vi "Teleop.vi"(10 "Match Info":T1={"Autonomous Elapsed Seconds"=0.0, "TeleOp Elapsed Seconds"=0.0, "Disabled Elapsed Seconds"=0.0, "Visited Autonomous"=FALSE, "Visited TeleOp"=FALSE, "Visited Disabled"=FALSE, "Autonomous Settings"={"Autonomous Style"=enum."Independent", "VI Refnum"=refnum}}, 11 "Call Context":T2) -> ()   [LabVIEW 2019]
doc: "This VI is called for each TeleOp packet received from the DS where the robot is not disabled. It is often used to read from the joysticks and update I/O or to update setpoints for timed control loops. It should complete and return within 20 milliseconds or it may miss DS packets."
uses:
  <vilib>/Rock Robotics/WPI/DriverStation/WPI_DriverStationDerivedRobotMode.ctl
  <vilib>/Rock Robotics/WPI/DriverStation/WPI_DriverStationMatch Info.ctl
  <vilib>/Rock Robotics/WPI/Utilities/WPI_GetSetVariantRefNum.vi
  Robot Global Data.vi
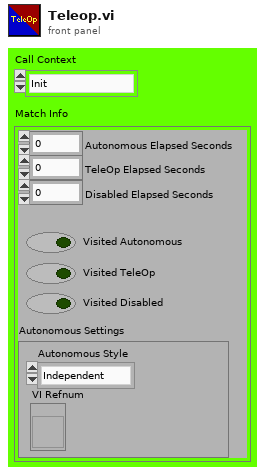
[diagram p1: front panel]
types:
  T1 = typedef "WPI_DriverStationMatch Info.ctl" = cluster{"Autonomous Elapsed Seconds":dbl, "TeleOp Elapsed Seconds":dbl, "Disabled Elapsed Seconds":dbl, "Visited Autonomous":bool, "Visited TeleOp":bool, "Visited Disabled":bool, "Autonomous Settings":cluster{"Autonomous Style":enum16{"Iterative", "Independent"}, "VI Refnum":refnum<vi>}}
  T2 = typedef "WPI_DriverStationDerivedRobotMode.ctl" = enum16{"Init", "Execute", "Stop"}
  T3 = typedef "WPI_JoystickDevRef.ctl" = cluster{"Device":T4}
  T4 = typedef "WPI_JoystickDeviceEnum.ctl" = enum16{"USB 0", "USB 1", "USB 2", "USB 3", "USB 4", "USB 5"}
  T5 = cluster{"Axes[0]":dbl, "Axes[1]":dbl, "Axes[2]":dbl, "Axes[3]":dbl, "Axes[4]":dbl, "Axes[5]":dbl, "Axes[6]":dbl, "Axes[7]":dbl}
  T6 = cluster{"Buttons[0]":bool, "Buttons[1]":bool, "Buttons[2]":bool, "Buttons[3]":bool, "Buttons[4]":bool, "Buttons[5]":bool, "Buttons[6]":bool, "Buttons[7]":bool, "Buttons[8]":bool, "Buttons[9]":bool, "Buttons[10]":bool, "Buttons[11]":bool, "Buttons[12]":bool, "Buttons[13]":bool, "Buttons[14]":bool, "Buttons[15]":bool, "Buttons[16]":bool, "Buttons[17]":bool, "Buttons[18]":bool, "Buttons[19]":bool, "Buttons[20]":bool, "Buttons[21]":bool, "Buttons[22]":bool, "Buttons[23]":bool, "Buttons[24]":bool, "Buttons[25]":bool, "Buttons[26]":bool, "Buttons[27]":bool, "Buttons[28]":bool, "Buttons[29]":bool, "Buttons[30]":bool, "Buttons[31]":bool, "Buttons[32]":bool, "Buttons[33]":bool, "Buttons[34]":bool, "Buttons[35]":bool, "Buttons[36]":bool, "Buttons[37]":bool, "Buttons[38]":bool, "Buttons[39]":bool, "Buttons[40]":bool, "Buttons[41]":bool, "Buttons[42]":bool, "Buttons[43]":bool, "Buttons[44]":bool, "Buttons[45]":bool, "Buttons[46]":bool, "Buttons[47]":bool, "Buttons[48]":bool, "Buttons[49]":bool}
  T7 = cluster{"POVs[0]":i16, "POVs[1]":i16, "POVs[2]":i16, "POVs[3]":i16, "POVs[4]":i16, "POVs[5]":i16, "POVs[6]":i16, "POVs[7]":i16, "POVs[8]":i16}
  T8 = cluster{"A1":dbl, "A2":dbl, "A3":dbl, "A4":dbl, "A5":dbl, "A6":dbl, "A7":dbl, "A8":dbl}
  T9 = cluster{"1":bool, "2":bool, "3":bool, "4":bool, "5":bool, "6":bool, "7":bool, "8":bool, "9":bool, "10":bool, "11":bool, "12":bool, "13":bool, "14":bool, "15":bool, "16":bool, "17":bool, "18":bool, "19":bool, "20":bool, "21":bool, "22":bool, "23":bool, "24":bool, "25":bool, "26":bool, "27":bool, "28":bool, "29":bool, "30":bool, "31":bool, "32":bool, "33":bool, "34":bool, "35":bool, "36":bool, "37":bool, "38":bool, "39":bool, "40":bool, "41":bool, "42":bool, "43":bool, "44":bool, "45":bool, "46":bool, "47":bool, "48":bool, "49":bool, "50":bool}
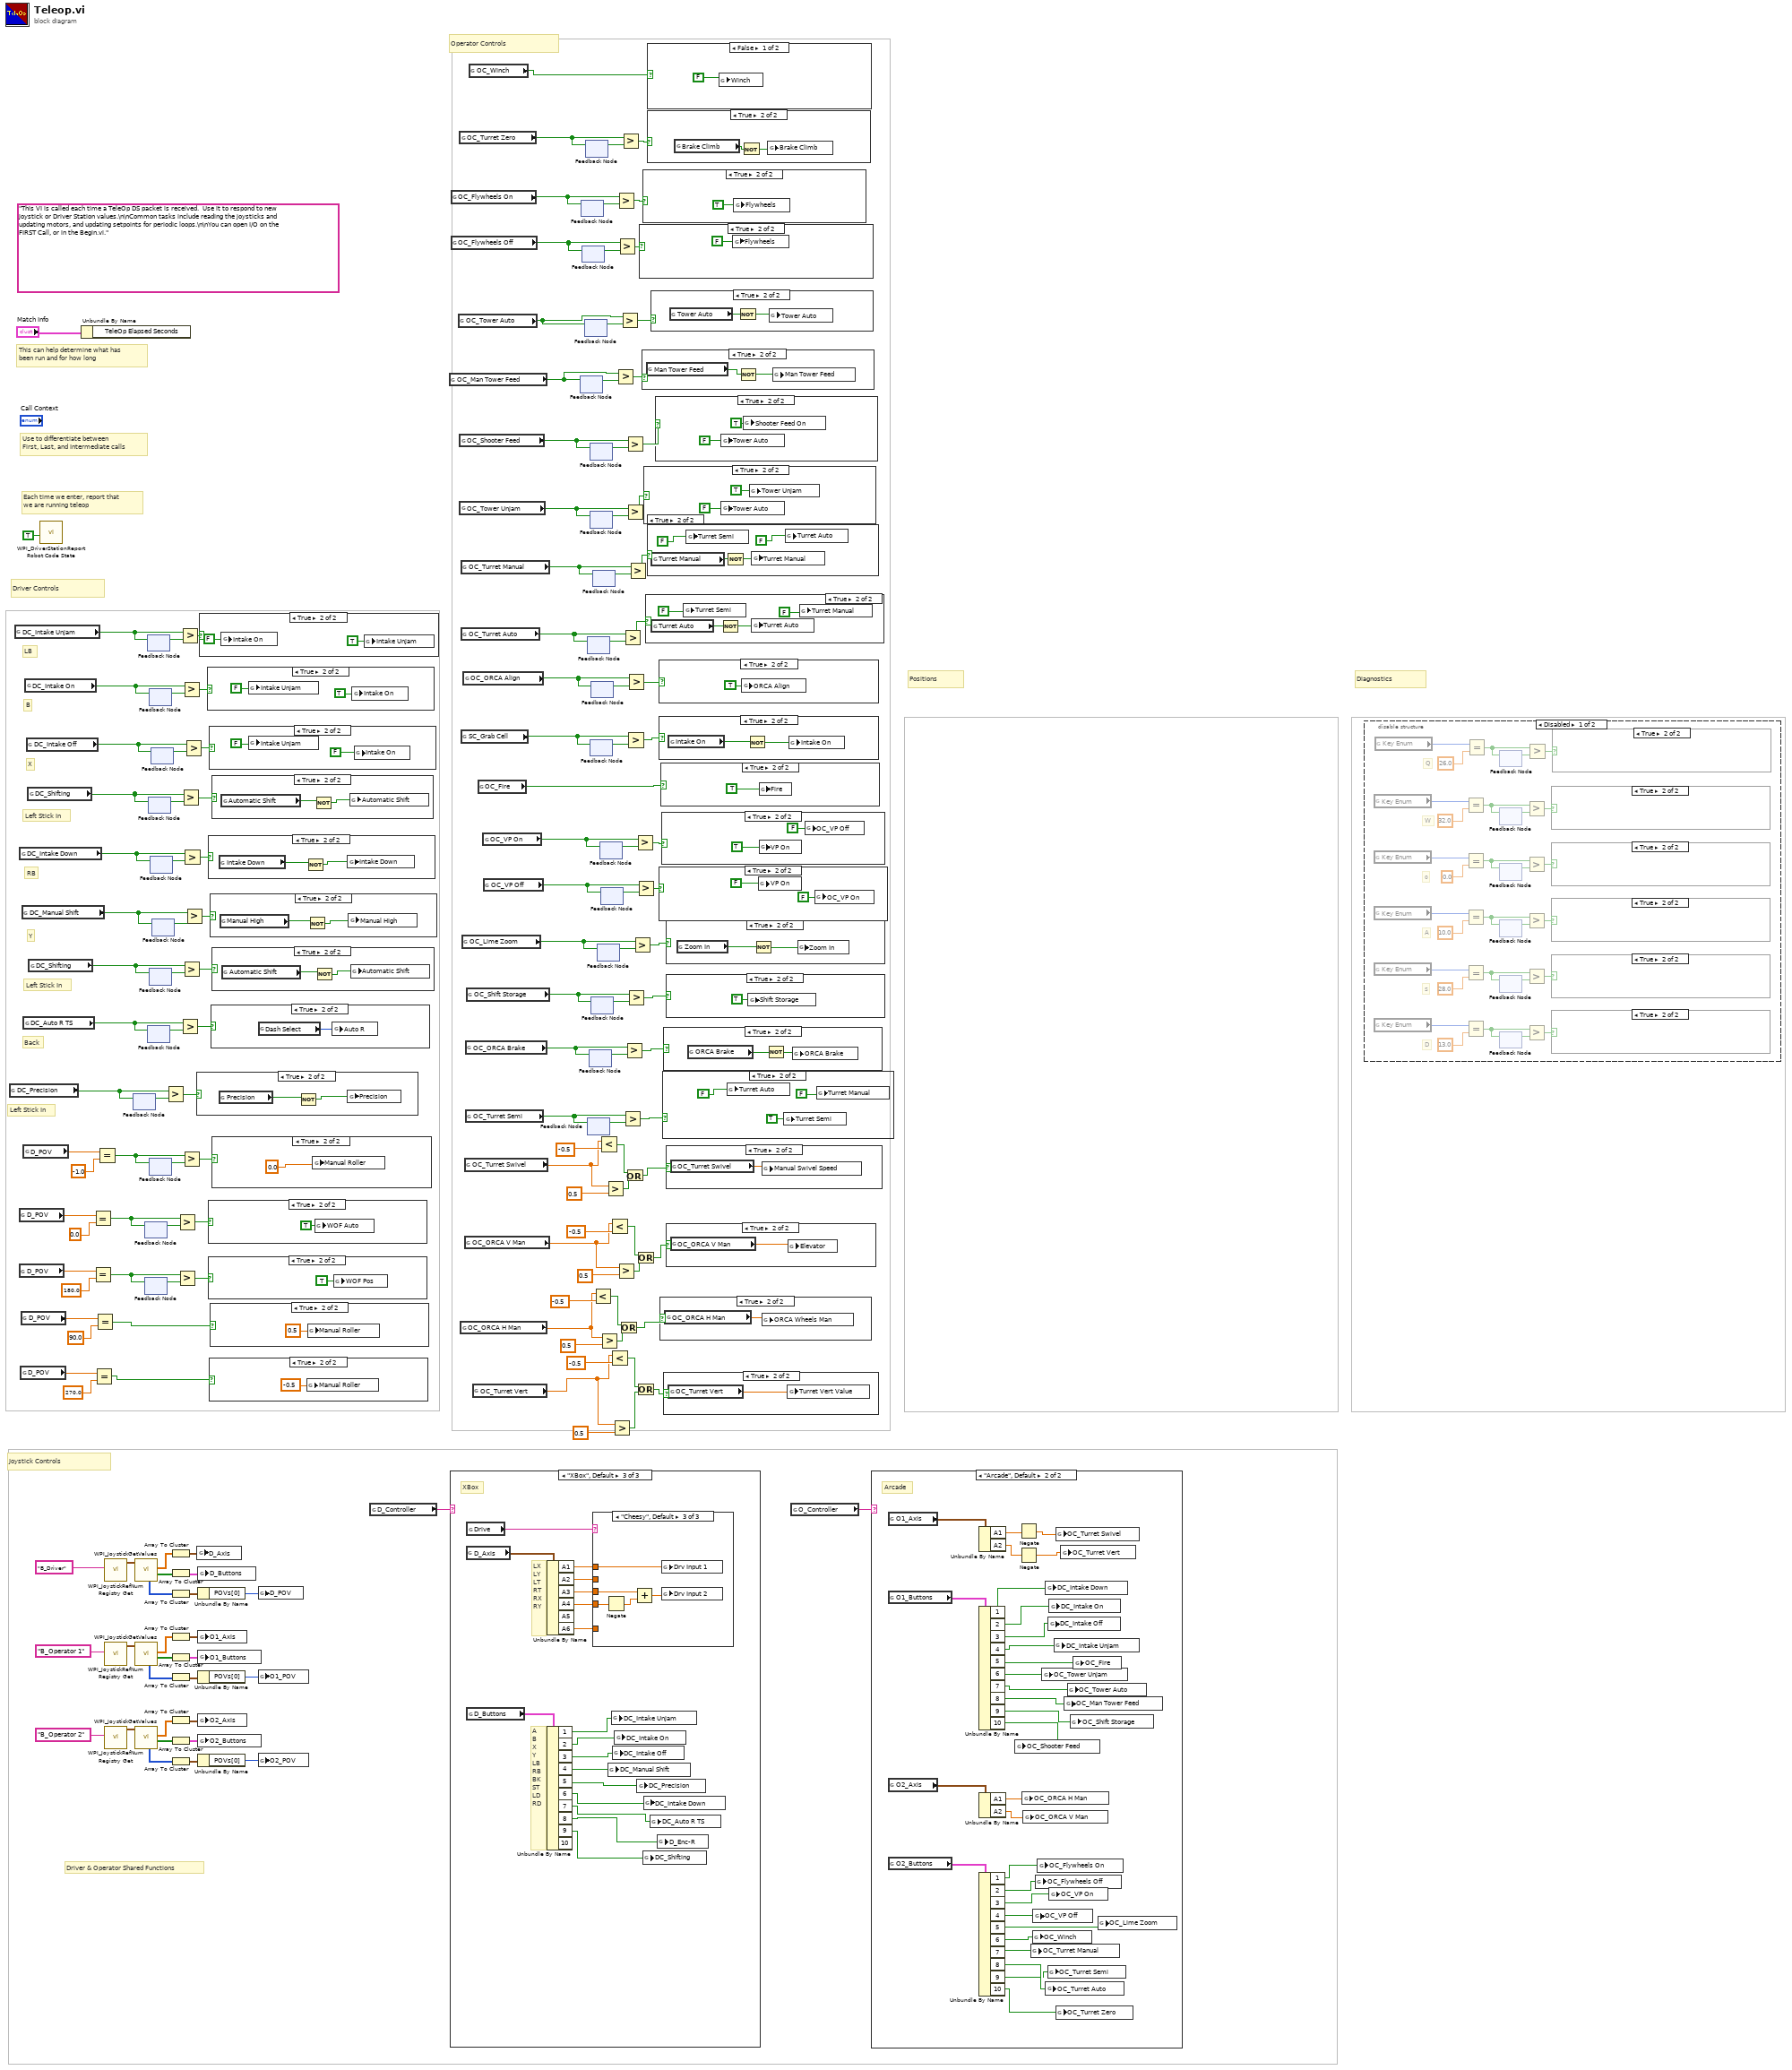
[diagram p0: block diagram]
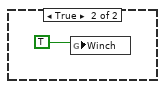
[diagram p2: hidden frame]
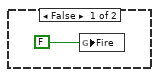
[diagram p7: hidden frame]
diagram:
  (unwired) "This VI is called each time a TeleOp DS packet is received.  Use it to respond to new joystick or Driver Station values.\n\nCommon tasks include reading the joysticks and updating motors, and updating setpoints for periodic loops.\n\nYou can open I/O on the FIRST Call, or in the Begin.vi."
  # "Left Stick In"
  # "B"
  # "X"
  # "Left Stick In"
  # "RB"
  # "Y"
  # "Left Stick In"
  # "Driver & Operator Shared Functions"
  # "Joystick Controls"
  # "Positions"
  # "Diagnostics"
  # "Operator Controls"
  # "Back"
  # "LB"
  # "Driver Controls"
  # "Each time we enter, report that\nwe are running teleop"
  # "Use to differentiate between\nFirst, Last, and Intermediate calls"
  # "This can help determine what has\nbeen run and for how long"
  n1 = global read "Robot Global Data.vi" "DC_Precision"() -> (w7:bool)
  n2 = global read "Robot Global Data.vi" "DC_Intake Unjam"() -> (w143:bool)
  n3 = global read "Robot Global Data.vi" "D_POV"() -> (w138:dbl)
  n4 = global read "Robot Global Data.vi" "D_POV"() -> (w148:dbl)
  n5 = global read "Robot Global Data.vi" "DC_Intake Down"() -> (w71:bool)
  n6 = global read "Robot Global Data.vi" "D_POV"() -> (w154:dbl)
  n7 = global read "Robot Global Data.vi" "D_POV"() -> (w84:dbl)
  n8 = global read "Robot Global Data.vi" "DC_Manual Shift"() -> (w76:bool)
  n9 = global read "Robot Global Data.vi" "DC_Auto R TS"() -> (w152:bool)
  n10 = global read "Robot Global Data.vi" "D_POV"() -> (w80:dbl)
  n11 = global read "Robot Global Data.vi" "DC_Intake On"() -> (w70:bool)
  n12 = global read "Robot Global Data.vi" "DC_Intake Off"() -> (w65:bool)
  n13 = global read "Robot Global Data.vi" "DC_Shifting"() -> (w64:bool)
  n14 = global read "Robot Global Data.vi" "DC_Shifting"() -> (w86:bool)
  n15 = call <vilib>:"WPI_DriverStationReport Robot Code State.vi"("TeleOp"=TRUE ("Autonomous")) -> ()  [unwired: 10 in, 1 out]
  n16 = Unbundle By Name("Match Info") -> ()  [unwired: 1 out]
  n17 = Equal?(x=w138, y=0.0) -> (x = y?=w144:bool)
  n18 = Equal?(x=w148, y=180.0) -> (x = y?=w145:bool)
  n19 = Equal?(x=w154, y=270.0) -> (x = y?=w83:bool)
  n20 = Equal?(x=w84, y=90.0) -> (x = y?=w82:bool)
  n21 = Equal?(x=w80, y=-1.0) -> (x = y?=w77:bool)
  n22 = call <vilib>:"WPI_JoystickRefNum Registry Get.vi"("refnum name"="B_Driver") -> ("JoystickDevRef"=w136:T3)  [unwired: 9 in, 1 out]
  n23 = call <vilib>:"WPI_JoystickRefNum Registry Get.vi"("refnum name"="B_Operator 1") -> ("JoystickDevRef"=w122:T3)  [unwired: 9 in, 1 out]
  n24 = call <vilib>:"WPI_JoystickRefNum Registry Get.vi"("refnum name"="B_Operator 2") -> ("JoystickDevRef"=w119:T3)  [unwired: 9 in, 1 out]
  n25 = feedback #1() -> (w5:bool)  [unwired: 1 in]
  n26 = feedback-in #1(w7) -> ()
  n27 = call <vilib>:"WPI_JoystickGetValues.vi"("JoystickDevRef"=w136) -> ("Buttons"=w134:bool[], "Axes"=w133:dbl[], "POVs"=w132:i16[])  [unwired: 6 in, 2 out]
  n28 = call <vilib>:"WPI_JoystickGetValues.vi"("JoystickDevRef"=w122) -> ("Buttons"=w124:bool[], "Axes"=w125:dbl[], "POVs"=w126:i16[])  [unwired: 6 in, 2 out]
  n29 = call <vilib>:"WPI_JoystickGetValues.vi"("JoystickDevRef"=w119) -> ("Buttons"=w117:bool[], "Axes"=w116:dbl[], "POVs"=w115:i16[])  [unwired: 6 in, 2 out]
  n30 = feedback #2() -> (w141:bool)  [unwired: 1 in]
  n31 = feedback-in #2(w144) -> ()
  n32 = feedback #3() -> (w147:bool)  [unwired: 1 in]
  n33 = feedback-in #3(w145) -> ()
  n34 = feedback #4() -> (w139:bool)  [unwired: 1 in]
  n35 = feedback-in #4(w143) -> ()
  n36 = feedback #5() -> (w150:bool)  [unwired: 1 in]
  n37 = feedback-in #5(w152) -> ()
  n38 = feedback #6() -> (w62:bool)  [unwired: 1 in]
  n39 = feedback-in #6(w64) -> ()
  n40 = feedback #7() -> (w68:bool)  [unwired: 1 in]
  n41 = feedback-in #7(w70) -> ()
  n42 = feedback #8() -> (w88:bool)  [unwired: 1 in]
  n43 = feedback-in #8(w86) -> ()
  n44 = feedback #9() -> (w79:bool)  [unwired: 1 in]
  n45 = feedback-in #9(w77) -> ()
  n46 = feedback #10() -> (w73:bool)  [unwired: 1 in]
  n47 = feedback-in #10(w71) -> ()
  n48 = feedback #11() -> (w67:bool)  [unwired: 1 in]
  n49 = feedback-in #11(w65) -> ()
  n50 = feedback #12() -> (w74:bool)  [unwired: 1 in]
  n51 = feedback-in #12(w76) -> ()
  n52 = Greater?(x=w7, y=w5) -> (0:w6:bool)
  n53 = Array To Cluster(array=w133) -> (cluster=w130:T5)
  n54 = Array To Cluster(array=w134) -> (cluster=w129:T6)
  n55 = Array To Cluster(array=w132) -> (cluster=w131:T7)
  n56 = Array To Cluster(array=w125) -> (cluster=w121:T5)
  n57 = Array To Cluster(array=w124) -> (cluster=w128:T6)
  n58 = Array To Cluster(array=w126) -> (cluster=w127:T7)
  n59 = Array To Cluster(array=w116) -> (cluster=w120:T5)
  n60 = Array To Cluster(array=w117) -> (cluster=w113:T6)
  n61 = Array To Cluster(array=w115) -> (cluster=w114:T7)
  n62 = Greater?(x=w144, y=w141) -> (0:w142:bool)
  n63 = Greater?(x=w145, y=w147) -> (0:w146:bool)
  n64 = Greater?(x=w143, y=w139) -> (0:w140:bool)
  n65 = Greater?(x=w152, y=w150) -> (0:w151:bool)
  n66 = Greater?(x=w64, y=w62) -> (0:w63:bool)
  n67 = Greater?(x=w70, y=w68) -> (0:w69:bool)
  n68 = Greater?(x=w86, y=w88) -> (0:w87:bool)
  n69 = Greater?(x=w77, y=w79) -> (0:w78:bool)
  n70 = Greater?(x=w71, y=w73) -> (0:w72:bool)
  n71 = Greater?(x=w65, y=w67) -> (0:w66:bool)
  n72 = Greater?(x=w76, y=w74) -> (0:w75:bool)
  n73 = case shown="True" w6 {
    frame False {
    }
    frame True {
      n74 = global read "Robot Global Data.vi" "Precision"() -> (w158:bool)
      n75 = Not(x=w158) -> (.not. x?=w157:bool)
      n76 = global write "Robot Global Data.vi" "Precision"(w157) -> ()
    }
  }
  n77 = global write "Robot Global Data.vi" "D_Axis"(w130) -> ()
  n78 = global write "Robot Global Data.vi" "D_Buttons"(w129) -> ()
  n79 = Unbundle By Name(w131) -> ("POVs[0]"=w112:i16)
  n80 = global write "Robot Global Data.vi" "O1_Axis"(w121) -> ()
  n81 = global write "Robot Global Data.vi" "O1_Buttons"(w128) -> ()
  n82 = Unbundle By Name(w127) -> ("POVs[0]"=w111:i16)
  n83 = global write "Robot Global Data.vi" "O2_Axis"(w120) -> ()
  n84 = global write "Robot Global Data.vi" "O2_Buttons"(w113) -> ()
  n85 = Unbundle By Name(w114) -> ("POVs[0]"=w110:i16)
  n86 = case shown="True" w140 {
    frame False {
    }
    frame True {
      n87 = global write "Robot Global Data.vi" "Intake On"(FALSE ("Intake On")) -> ()
      n88 = global write "Robot Global Data.vi" "Intake Unjam"(TRUE ("Intake Unjam")) -> ()
    }
  }
  n89 = case shown="True" w69 {
    frame False {
    }
    frame True {
      n90 = global write "Robot Global Data.vi" "Intake Unjam"(FALSE ("Intake On")) -> ()
      n91 = global write "Robot Global Data.vi" "Intake On"(TRUE ("Intake On")) -> ()
    }
  }
  n92 = case shown="True" w72 {
    frame False {
    }
    frame True {
      n93 = global read "Robot Global Data.vi" "Intake Down"() -> (w164:bool)
      n94 = Not(x=w164) -> (.not. x?=w163:bool)
      n95 = global write "Robot Global Data.vi" "Intake Down"(w163) -> ()
    }
  }
  n96 = case shown="True" w142 {
    frame False {
    }
    frame True {
      n97 = global write "Robot Global Data.vi" "WOF Auto"(TRUE ("DC_WOF")) -> ()
    }
  }
  n98 = case shown="True" w146 {
    frame False {
    }
    frame True {
      n99 = global write "Robot Global Data.vi" "WOF Pos"(TRUE ("WOF Pos")) -> ()
    }
  }
  n100 = case shown="True" w66 {
    frame False {
    }
    frame True {
      n101 = global write "Robot Global Data.vi" "Intake Unjam"(FALSE ("Intake On")) -> ()
      n102 = global write "Robot Global Data.vi" "Intake On"(FALSE ("Manual High")) -> ()
    }
  }
  n103 = case shown="True" w83 {
    frame False {
    }
    frame True {
      n104 = global write "Robot Global Data.vi" "Manual Roller"(-0.5 ("Manual Roller")) -> ()
    }
  }
  n105 = case shown="True" w75 {
    frame False {
    }
    frame True {
      n106 = global read "Robot Global Data.vi" "Manual High"() -> (w171:bool)
      n107 = Not(x=w171) -> (.not. x?=w170:bool)
      n108 = global write "Robot Global Data.vi" "Manual High"(w170) -> ()
    }
  }
  n109 = case shown="True" w82 {
    frame False {
    }
    frame True {
      n110 = global write "Robot Global Data.vi" "Manual Roller"(0.5 ("Manual Roller")) -> ()
    }
  }
  n111 = case shown="True" w151 {
    frame False {
    }
    frame True {
      n112 = global read "Robot Global Data.vi" "Dash Select"() -> (w173:i8)
      n113 = global write "Robot Global Data.vi" "Auto R"(w173) -> ()
    }
  }
  n114 = case shown="True" w63 {
    frame False {
    }
    frame True {
      n115 = global read "Robot Global Data.vi" "Automatic Shift"() -> (w175:bool)
      n116 = Not(x=w175) -> (.not. x?=w174:bool)
      n117 = global write "Robot Global Data.vi" "Automatic Shift"(w174) -> ()
    }
  }
  n118 = case shown="True" w87 {
    frame False {
    }
    frame True {
      n119 = global read "Robot Global Data.vi" "Automatic Shift"() -> (w177:bool)
      n120 = Not(x=w177) -> (.not. x?=w176:bool)
      n121 = global write "Robot Global Data.vi" "Automatic Shift"(w176) -> ()
    }
  }
  n122 = case shown="True" w78 {
    frame False {
    }
    frame True {
      n123 = global write "Robot Global Data.vi" "Manual Roller"(0.0 ("Manual Roller")) -> ()
    }
  }
  n124 = global write "Robot Global Data.vi" "D_POV"(w112) -> ()
  n125 = global write "Robot Global Data.vi" "O1_POV"(w111) -> ()
  n126 = global write "Robot Global Data.vi" "O2_POV"(w110) -> ()
  n127 = global read "Robot Global Data.vi" "D_Controller"() -> (w109:string)
  n128 = global read "Robot Global Data.vi" "OC_Man Tower Feed"() -> (w3:bool)
  n129 = case shown="\"XBox\", Default" w109 {
    frame "Sticks" {
    }
    frame "Steering" {
    }
    frame "XBox", Default {
      # "LX\nLY\nLT\nRT\nRX\nRY"
      # "A\nB\nX\nY\nLB\nRB\nBK\nST\nLD\nRD"
      # "XBox"
      n130 = global read "Robot Global Data.vi" "D_Axis"() -> (w195:T8)
      n131 = global read "Robot Global Data.vi" "Drive"() -> (w194:string)
      n132 = global read "Robot Global Data.vi" "D_Buttons"() -> (w188:T9)
      n133 = Unbundle By Name(w195) -> ("A1"=w193:dbl, "A2"=w190:dbl, "A3"=w192:dbl, "A4"=w191:dbl, "A6"=w189:dbl)  [unwired: 1 out]
      n134 = Unbundle By Name(w188) -> ("1"=w181:bool, "2"=w182:bool, "3"=w183:bool, "4"=w185:bool, "5"=w187:bool, "6"=w184:bool, "7"=w179:bool, "8"=w180:bool, "9"=w186:bool)  [unwired: 1 out]
      n135 = case shown="\"Cheesy\", Default" w194 {
        tunnel: w193 -> [_ w199 w204]
        tunnel: w192 -> [_ _ w203]
        tunnel: w191 -> [_ _ w202]
        tunnel: w190 -> [w197 w198 _]
        tunnel: w189 -> [w196 _ _]
        frame "Tank" {
          n136 = global write "Robot Global Data.vi" "Drv Input 1"(w197) -> ()
          n137 = global write "Robot Global Data.vi" "Drv Input 2"(w196) -> ()
        }
        frame "Arcade" {
          n138 = Multiply(x=w198, y=-1.0) -> (x*y=w200:dbl)
          n139 = global write "Robot Global Data.vi" "Drv Input 1"(w199) -> ()
          n140 = global write "Robot Global Data.vi" "Drv Input 2"(w200) -> ()
        }
        frame "Cheesy", Default {
          n141 = Negate(x=w202) -> (-x=w206:dbl)
          n142 = Add(x=w203, y=w206) -> (x+y=w205:dbl)
          n143 = global write "Robot Global Data.vi" "Drv Input 1"(w204) -> ()
          n144 = global write "Robot Global Data.vi" "Drv Input 2"(w205) -> ()
        }
      }
      n145 = global write "Robot Global Data.vi" "DC_Manual Shift"(w185) -> ()
      n146 = global write "Robot Global Data.vi" "DC_Intake Unjam"(w181) -> ()
      n147 = global write "Robot Global Data.vi" "DC_Intake Off"(w183) -> ()
      n148 = global write "Robot Global Data.vi" "DC_Intake On"(w182) -> ()
      n149 = global write "Robot Global Data.vi" "DC_Precision"(w187) -> ()
      n150 = global write "Robot Global Data.vi" "DC_Shifting"(w186) -> ()
      n151 = global write "Robot Global Data.vi" "DC_Intake Down"(w184) -> ()
      n152 = global write "Robot Global Data.vi" "DC_Auto R TS"(w179) -> ()
      n153 = global write "Robot Global Data.vi" "D_Enc-R"(w180) -> ()
    }
  }
  n154 = global read "Robot Global Data.vi" "OC_Flywheels On"() -> (w15:bool)
  n155 = global read "Robot Global Data.vi" "OC_Flywheels Off"() -> (w12:bool)
  n156 = global read "Robot Global Data.vi" "OC_Tower Auto"() -> (w45:bool)
  n157 = global read "Robot Global Data.vi" "OC_Turret Zero"() -> (w9:bool)
  n158 = global read "Robot Global Data.vi" "OC_Shooter Feed"() -> (w58:bool)
  n159 = global read "Robot Global Data.vi" "OC_Tower Unjam"() -> (w59:bool)
  n160 = global read "Robot Global Data.vi" "OC_ORCA H Man"() -> (w22:dbl)
  n161 = global read "Robot Global Data.vi" "OC_Turret Manual"() -> (w92:bool)
  n162 = global read "Robot Global Data.vi" "OC_Turret Auto"() -> (w93:bool)
  n163 = global read "Robot Global Data.vi" "SC_Grab Cell"() -> (w102:bool)
  n164 = global read "Robot Global Data.vi" "OC_Lime Zoom"() -> (w49:bool)
  n165 = global read "Robot Global Data.vi" "OC_ORCA Align"() -> (w106:bool)
  n166 = global read "Robot Global Data.vi" "OC_Turret Swivel"() -> (w43:dbl)
  n167 = global read "Robot Global Data.vi" "OC_ORCA V Man"() -> (w29:dbl)
  n168 = global read "Robot Global Data.vi" "OC_ORCA Brake"() -> (w95:bool)
  n169 = global read "Robot Global Data.vi" "OC_Turret Semi"() -> (w20:bool)
  n170 = global read "Robot Global Data.vi" "OC_Shift Storage"() -> (w100:bool)
  n171 = global read "Robot Global Data.vi" "OC_Winch"() -> (w1:bool)
  n172 = global read "Robot Global Data.vi" "OC_Turret Vert"() -> (w35:dbl)
  n173 = global read "Robot Global Data.vi" "OC_Fire"() -> (w17:bool)
  n174 = global read "Robot Global Data.vi" "OC_VP On"() -> (w54:bool)
  n175 = global read "Robot Global Data.vi" "OC_VP Off"() -> (w51:bool)
  n176 = feedback #13() -> (w4:bool)  [unwired: 1 in]
  n177 = feedback-in #13(w3) -> ()
  n178 = feedback #14() -> (w16:bool)  [unwired: 1 in]
  n179 = feedback-in #14(w15) -> ()
  n180 = feedback #15() -> (w11:bool)  [unwired: 1 in]
  n181 = feedback-in #15(w12) -> ()
  n182 = feedback #16() -> (w46:bool)  [unwired: 1 in]
  n183 = feedback-in #16(w45) -> ()
  n184 = feedback #17() -> (w8:bool)  [unwired: 1 in]
  n185 = feedback-in #17(w9) -> ()
  n186 = feedback #18() -> (w94:bool)  [unwired: 1 in]
  n187 = feedback-in #18(w93) -> ()
  n188 = feedback #19() -> (w18:bool)  [unwired: 1 in]
  n189 = feedback-in #19(w20) -> ()
  n190 = feedback #20() -> (w97:bool)  [unwired: 1 in]
  n191 = feedback-in #20(w95) -> ()
  n192 = feedback #21() -> (w57:bool)  [unwired: 1 in]
  n193 = feedback-in #21(w58) -> ()
  n194 = feedback #22() -> (w60:bool)  [unwired: 1 in]
  n195 = feedback-in #22(w59) -> ()
  n196 = feedback #23() -> (w104:bool)  [unwired: 1 in]
  n197 = feedback-in #23(w102) -> ()
  n198 = feedback #24() -> (w105:bool)  [unwired: 1 in]
  n199 = feedback-in #24(w106) -> ()
  n200 = feedback #25() -> (w98:bool)  [unwired: 1 in]
  n201 = feedback-in #25(w100) -> ()
  n202 = Less?(x=w22, y=-0.5) -> (x < y?=w25:bool)
  n203 = feedback #26() -> (w91:bool)  [unwired: 1 in]
  n204 = feedback-in #26(w92) -> ()
  n205 = feedback #27() -> (w47:bool)  [unwired: 1 in]
  n206 = feedback-in #27(w49) -> ()
  n207 = Less?(x=w43, y=-0.5) -> (x < y?=w41:bool)
  n208 = Greater?(x=w22, y=0.5) -> (0:w26:bool)
  n209 = feedback #28() -> (w55:bool)  [unwired: 1 in]
  n210 = feedback-in #28(w54) -> ()
  n211 = feedback #29() -> (w50:bool)  [unwired: 1 in]
  n212 = feedback-in #29(w51) -> ()
  n213 = Greater?(x=w43, y=0.5) -> (0:w42:bool)
  n214 = Less?(x=w29, y=-0.5) -> (x < y?=w31:bool)
  n215 = Less?(x=w35, y=-0.5) -> (x < y?=w36:bool)
  n216 = Greater?(x=w35, y=0.5) -> (0:w37:bool)
  n217 = Greater?(x=w3, y=w4) -> (0:w2:bool)
  n218 = Greater?(x=w15, y=w16) -> (0:w14:bool)
  n219 = Greater?(x=w29, y=0.5) -> (0:w32:bool)
  n220 = Greater?(x=w12, y=w11) -> (0:w13:bool)
  n221 = Or(x=w25, y=w26) -> (x .or. y?=w24:bool)
  n222 = Greater?(x=w45, y=w46) -> (0:w21:bool)
  n223 = Greater?(x=w9, y=w8) -> (0:w10:bool)
  n224 = Greater?(x=w93, y=w94) -> (0:w90:bool)
  n225 = Greater?(x=w20, y=w18) -> (0:w19:bool)
  n226 = Greater?(x=w95, y=w97) -> (0:w96:bool)
  n227 = Greater?(x=w58, y=w57) -> (0:w56:bool)
  n228 = Greater?(x=w59, y=w60) -> (0:w61:bool)
  n229 = Or(x=w41, y=w42) -> (x .or. y?=w40:bool)
  n230 = Greater?(x=w102, y=w104) -> (0:w103:bool)
  n231 = Greater?(x=w106, y=w105) -> (0:w107:bool)
  n232 = Greater?(x=w100, y=w98) -> (0:w99:bool)
  n233 = Greater?(x=w92, y=w91) -> (0:w89:bool)
  n234 = Greater?(x=w49, y=w47) -> (0:w48:bool)
  n235 = Greater?(x=w54, y=w55) -> (0:w53:bool)
  n236 = Greater?(x=w51, y=w50) -> (0:w52:bool)
  n237 = Or(x=w31, y=w32) -> (x .or. y?=w28:bool)
  n238 = Or(x=w36, y=w37) -> (x .or. y?=w34:bool)
  n239 = case shown="True" w13 {
    frame False {
    }
    frame True {
      n240 = global write "Robot Global Data.vi" "Flywheels"(FALSE ("High Gear")) -> ()
    }
  }
  n241 = case shown="True" w2 {
    frame False {
    }
    frame True {
      n242 = global read "Robot Global Data.vi" "Man Tower Feed"() -> (w208:bool)
      n243 = Not(x=w208) -> (.not. x?=w209:bool)
      n244 = global write "Robot Global Data.vi" "Man Tower Feed"(w209) -> ()
    }
  }
  n245 = case shown="True" w14 {
    frame False {
    }
    frame True {
      n246 = global write "Robot Global Data.vi" "Flywheels"(TRUE ("High Gear")) -> ()
    }
  }
  n247 = case shown="True" w61 {
    frame False {
    }
    frame True {
      n248 = global write "Robot Global Data.vi" "Tower Auto"(FALSE ("Turret Manual")) -> ()
      n249 = global write "Robot Global Data.vi" "Tower Unjam"(TRUE ("Turret Manual")) -> ()
    }
  }
  n250 = case shown="True" w90 {
    frame False {
    }
    frame True {
      n251 = global read "Robot Global Data.vi" "Turret Auto"() -> (w216:bool)
      n252 = global write "Robot Global Data.vi" "Turret Semi"(FALSE) -> ()
      n253 = Not(x=w216) -> (.not. x?=w215:bool)
      n254 = global write "Robot Global Data.vi" "Turret Auto"(w215) -> ()
      n255 = global write "Robot Global Data.vi" "Turret Manual"(FALSE) -> ()
    }
  }
  n256 = case shown="True" w10 {
    frame False {
    }
    frame True {
      n257 = global read "Robot Global Data.vi" "Brake Climb"() -> (w218:bool)
      n258 = Not(x=w218) -> (.not. x?=w217:bool)
      n259 = global write "Robot Global Data.vi" "Brake Climb"(w217) -> ()
    }
  }
  n260 = case shown="True" w89 {
    frame False {
    }
    frame True {
      n261 = global read "Robot Global Data.vi" "Turret Manual"() -> (w222:bool)
      n262 = global write "Robot Global Data.vi" "Turret Semi"(FALSE) -> ()
      n263 = Not(x=w222) -> (.not. x?=w221:bool)
      n264 = global write "Robot Global Data.vi" "Turret Manual"(w221) -> ()
      n265 = global write "Robot Global Data.vi" "Turret Auto"(FALSE) -> ()
    }
  }
  n266 = case shown="False" w1 {
    frame False {
      n267 = global write "Robot Global Data.vi" "Winch"(FALSE ("Winch")) -> ()
    }
    frame True {
      n268 = global write "Robot Global Data.vi" "Winch"(TRUE ("Winch")) -> ()
    }
  }
  n269 = case shown="True" w21 {
    frame False {
    }
    frame True {
      n270 = global read "Robot Global Data.vi" "Tower Auto"() -> (w226:bool)
      n271 = Not(x=w226) -> (.not. x?=w225:bool)
      n272 = global write "Robot Global Data.vi" "Tower Auto"(w225) -> ()
    }
  }
  n273 = case shown="True" w56 {
    frame False {
    }
    frame True {
      n274 = global write "Robot Global Data.vi" "Tower Auto"(FALSE ("Turret Manual")) -> ()
      n275 = global write "Robot Global Data.vi" "Shooter Feed On"(TRUE ("Turret Manual")) -> ()
    }
  }
  n276 = case shown="True" w52 {
    frame False {
    }
    frame True {
      n277 = global write "Robot Global Data.vi" "VP On"(FALSE ("High Gear")) -> ()
      n278 = global write "Robot Global Data.vi" "OC_VP On"(FALSE ("OC_VP On")) -> ()
    }
  }
  n279 = case shown="True" w107 {
    frame False {
    }
    frame True {
      n280 = global write "Robot Global Data.vi" "ORCA Align"(TRUE ("High Gear")) -> ()
    }
  }
  n281 = case shown="True" w103 {
    frame False {
    }
    frame True {
      n282 = global read "Robot Global Data.vi" "Intake On"() -> (w233:bool)
      n283 = Not(x=w233) -> (.not. x?=w232:bool)
      n284 = global write "Robot Global Data.vi" "Intake On"(w232) -> ()
    }
  }
  n285 = case shown="True" w24 {
    frame False {
      n286 = global write "Robot Global Data.vi" "ORCA Wheels Man"(0.0 ("ORCA Wheels Man")) -> ()
    }
    frame True {
      n287 = global read "Robot Global Data.vi" "OC_ORCA H Man"() -> (w235:dbl)
      n288 = global write "Robot Global Data.vi" "ORCA Wheels Man"(w235) -> ()
    }
  }
  n289 = case shown="True" w17 {
    frame False {
      n290 = global write "Robot Global Data.vi" "Fire"(FALSE ("High Gear")) -> ()
    }
    frame True {
      n291 = global write "Robot Global Data.vi" "Fire"(TRUE ("High Gear")) -> ()
    }
  }
  n292 = case shown="True" w53 {
    frame False {
    }
    frame True {
      n293 = global write "Robot Global Data.vi" "VP On"(TRUE ("High Gear")) -> ()
      n294 = global write "Robot Global Data.vi" "OC_VP Off"(FALSE ("OC_VP On")) -> ()
    }
  }
  n295 = case shown="True" w19 {
    frame False {
    }
    frame True {
      n296 = global write "Robot Global Data.vi" "Turret Auto"(FALSE) -> ()
      n297 = global write "Robot Global Data.vi" "Turret Semi"(TRUE ("Turret Semi")) -> ()
      n298 = global write "Robot Global Data.vi" "Turret Manual"(FALSE) -> ()
    }
  }
  n299 = case shown="True" w96 {
    frame False {
    }
    frame True {
      n300 = global read "Robot Global Data.vi" "ORCA Brake"() -> (w243:bool)
      n301 = Not(x=w243) -> (.not. x?=w244:bool)
      n302 = global write "Robot Global Data.vi" "ORCA Brake"(w244) -> ()
    }
  }
  n303 = case shown="True" w34 {
    frame False {
      n304 = global write "Robot Global Data.vi" "Turret Vert Value"(0.0 ("Turret Vert Value")) -> ()
    }
    frame True {
      n305 = global read "Robot Global Data.vi" "OC_Turret Vert"() -> (w246:dbl)
      n306 = global write "Robot Global Data.vi" "Turret Vert Value"(w246) -> ()
    }
  }
  n307 = case shown="True" w48 {
    frame False {
    }
    frame True {
      n308 = global read "Robot Global Data.vi" "Zoom In"() -> (w248:bool)
      n309 = Not(x=w248) -> (.not. x?=w247:bool)
      n310 = global write "Robot Global Data.vi" "Zoom In"(w247) -> ()
    }
  }
  n311 = case shown="True" w99 {
    frame False {
    }
    frame True {
      n312 = global write "Robot Global Data.vi" "Shift Storage"(TRUE ("Cargo Latch")) -> ()
    }
  }
  n313 = case shown="True" w40 {
    frame False {
      n314 = global write "Robot Global Data.vi" "Manual Swivel Speed"(0.0 ("Manual Swivel Speed")) -> ()
    }
    frame True {
      n315 = global read "Robot Global Data.vi" "OC_Turret Swivel"() -> (w251:dbl)
      n316 = global write "Robot Global Data.vi" "Manual Swivel Speed"(w251) -> ()
    }
  }
  n317 = case shown="True" w28 {
    frame False {
      n318 = global write "Robot Global Data.vi" "Elevator"(0.0 ("Elevator")) -> ()
    }
    frame True {
      n319 = global read "Robot Global Data.vi" "OC_ORCA V Man"() -> (w253:dbl)
      n320 = global write "Robot Global Data.vi" "Elevator"(w253) -> ()
    }
  }
  n321 = global read "Robot Global Data.vi" "O_Controller"() -> (w108:string)
  n322 = case shown="\"Arcade\", Default" w108 {
    frame "XBox" {
      # "LX\nLY\nLT\nRT\nRX\nRY"
      # "A\nB\nX\nY\nLB\nRB\nBK\nST\nLD\nRD"
      # "XBox"
      n323 = global read "Robot Global Data.vi" "O1_Axis"() -> (w262:T8)
      n324 = global read "Robot Global Data.vi" "O1_Buttons"() -> (w263:T9)
      n325 = Unbundle By Name(w262) -> ("A1"=w261:dbl, "A4"=w259:dbl, "A5"=w257:dbl, "A6"=w256:dbl)  [unwired: 2 out]
      n326 = Unbundle By Name(w263) -> ("2"=w254:bool, "4"=w260:bool, "5"=w255:bool, "6"=w258:bool)  [unwired: 6 out]
      n327 = global write "Robot Global Data.vi" "OC_Turret Swivel"(w261) -> ()
      n328 = global write "Robot Global Data.vi" "OC_ORCA H Man"(w257) -> ()
      n329 = global write "Robot Global Data.vi" "OC_ORCA V Man"(w256) -> ()
      n330 = global write "Robot Global Data.vi" "OC_Turret"(w259) -> ()
      n331 = global write "Robot Global Data.vi" "OC_Shift Storage"(w255) -> ()
      n332 = global write "Robot Global Data.vi" "OC_ORCA Brake"(w254) -> ()
      n333 = global write "Robot Global Data.vi" "OC_ORCA Align"(w258) -> ()
      n334 = global write "Robot Global Data.vi" "SC_Grab Cell"(w260) -> ()
    }
    frame "Arcade", Default {
      # "Arcade"
      n335 = global read "Robot Global Data.vi" "O1_Axis"() -> (w293:T8)
      n336 = global read "Robot Global Data.vi" "O1_Buttons"() -> (w292:T9)
      n337 = global read "Robot Global Data.vi" "O2_Axis"() -> (w290:T8)
      n338 = global read "Robot Global Data.vi" "O2_Buttons"() -> (w291:T9)
      n339 = Unbundle By Name(w293) -> ("A1"=w271:dbl, "A2"=w268:dbl)
      n340 = Unbundle By Name(w290) -> ("A1"=w289:dbl, "A2"=w288:dbl)
      n341 = Unbundle By Name(w292) -> ("1"=w286:bool, "2"=w285:bool, "3"=w284:bool, "4"=w283:bool, "5"=w274:bool, "6"=w278:bool, "7"=w276:bool, "8"=w277:bool, "9"=w275:bool, "10"=w282:bool)
      n342 = Unbundle By Name(w291) -> ("1"=w273:bool, "2"=w272:bool, "3"=w281:bool, "4"=w280:bool, "5"=w279:bool, "6"=w264:bool, "7"=w287:bool, "8"=w266:bool, "9"=w265:bool, "10"=w267:bool)
      n343 = global write "Robot Global Data.vi" "OC_Shooter Feed"(w282) -> ()
      n344 = Negate(x=w271) -> (-x=w270:dbl)
      n345 = Negate(x=w268) -> (-x=w269:dbl)
      n346 = global write "Robot Global Data.vi" "OC_ORCA H Man"(w289) -> ()
      n347 = global write "Robot Global Data.vi" "OC_ORCA V Man"(w288) -> ()
      n348 = global write "Robot Global Data.vi" "OC_Turret Manual"(w287) -> ()
      n349 = global write "Robot Global Data.vi" "OC_Winch"(w264) -> ()
      n350 = global write "Robot Global Data.vi" "OC_VP Off"(w280) -> ()
      n351 = global write "Robot Global Data.vi" "OC_Flywheels Off"(w272) -> ()
      n352 = global write "Robot Global Data.vi" "OC_Flywheels On"(w273) -> ()
      n353 = global write "Robot Global Data.vi" "OC_Tower Unjam"(w278) -> ()
      n354 = global write "Robot Global Data.vi" "DC_Intake Down"(w286) -> ()
      n355 = global write "Robot Global Data.vi" "OC_Turret Auto"(w266) -> ()
      n356 = global write "Robot Global Data.vi" "OC_Turret Semi"(w265) -> ()
      n357 = global write "Robot Global Data.vi" "DC_Intake Off"(w284) -> ()
      n358 = global write "Robot Global Data.vi" "DC_Intake On"(w285) -> ()
      n359 = global write "Robot Global Data.vi" "OC_VP On"(w281) -> ()
      n360 = global write "Robot Global Data.vi" "DC_Intake Unjam"(w283) -> ()
      n361 = global write "Robot Global Data.vi" "OC_Turret Swivel"(w270) -> ()
      n362 = global write "Robot Global Data.vi" "OC_Turret Zero"(w267) -> ()
      n363 = global write "Robot Global Data.vi" "OC_Turret Vert"(w269) -> ()
      n364 = global write "Robot Global Data.vi" "OC_Man Tower Feed"(w277) -> ()
      n365 = global write "Robot Global Data.vi" "OC_Tower Auto"(w276) -> ()
      n366 = global write "Robot Global Data.vi" "OC_Shift Storage"(w275) -> ()
      n367 = global write "Robot Global Data.vi" "OC_Fire"(w274) -> ()
      n368 = global write "Robot Global Data.vi" "OC_Lime Zoom"(w279) -> ()
    }
  }
  n369 = disable-structure shown="Disabled" {
    frame Disabled {
      # "A"
      # "D"
      # "S"
      # "0"
      # "W"
      # "Q"
      n370 = global read "Robot Global Data.vi" "Key Enum"() -> (w321:i16)
      n371 = global read "Robot Global Data.vi" "Key Enum"() -> (w318:i16)
      n372 = global read "Robot Global Data.vi" "Key Enum"() -> (w298:i16)
      n373 = global read "Robot Global Data.vi" "Key Enum"() -> (w316:i16)
      n374 = global read "Robot Global Data.vi" "Key Enum"() -> (w315:i16)
      n375 = global read "Robot Global Data.vi" "Key Enum"() -> (w322:i16)
      n376 = Equal?(x=w321, y=32.0) -> (x = y?=w302:bool)
      n377 = Equal?(x=w318, y=0.0) -> (x = y?=w301:bool)
      n378 = Equal?(x=w298, y=10.0) -> (x = y?=w294:bool)
      n379 = Equal?(x=w316, y=28.0) -> (x = y?=w300:bool)
      n380 = Equal?(x=w315, y=13.0) -> (x = y?=w299:bool)
      n381 = Equal?(x=w322, y=26.0) -> (x = y?=w303:bool)
      n382 = feedback #30() -> (w307:bool)  [unwired: 1 in]
      n383 = feedback-in #30(w302) -> ()
      n384 = feedback #31() -> (w308:bool)  [unwired: 1 in]
      n385 = feedback-in #31(w301) -> ()
      n386 = feedback #32() -> (w296:bool)  [unwired: 1 in]
      n387 = feedback-in #32(w294) -> ()
      n388 = feedback #33() -> (w310:bool)  [unwired: 1 in]
      n389 = feedback-in #33(w300) -> ()
      n390 = feedback #34() -> (w313:bool)  [unwired: 1 in]
      n391 = feedback-in #34(w299) -> ()
      n392 = feedback #35() -> (w304:bool)  [unwired: 1 in]
      n393 = feedback-in #35(w303) -> ()
      n394 = Greater?(x=w302, y=w307) -> (0:w306:bool)
      n395 = Greater?(x=w301, y=w308) -> (0:w309:bool)
      n396 = Greater?(x=w294, y=w296) -> (0:w295:bool)
      n397 = Greater?(x=w300, y=w310) -> (0:w311:bool)
      n398 = Greater?(x=w299, y=w313) -> (0:w312:bool)
      n399 = Greater?(x=w303, y=w304) -> (0:w305:bool)
      n400 = case shown="True" w306 {
        frame False {
        }
        frame True {
        }
      }
      n401 = case shown="True" w309 {
        frame False {
        }
        frame True {
        }
      }
      n402 = case shown="True" w295 {
        frame False {
        }
        frame True {
        }
      }
      n403 = case shown="True" w311 {
        frame False {
        }
        frame True {
        }
      }
      n404 = case shown="True" w312 {
        frame False {
        }
        frame True {
        }
      }
      n405 = case shown="True" w305 {
        frame False {
        }
        frame True {
        }
      }
    }
    frame Enabled {
    }
  }
